vi "plane_from_3-pts.vi"(11 "Input":dbl[][](array[numeric])) -> (2 "Cross Product":dbl[](array[numeric]), 3 "gradient-out":dbl[](array[numeric]))   [LabVIEW 2024]
uses:
  <vilib>/Analysis/NI_AALPro.lvlib
panel:
  out "element":dbl
  out "In 3":dbl[](array[numeric])
  out "In 2":dbl[](array[numeric])
  out "In 1":dbl[](array[numeric])
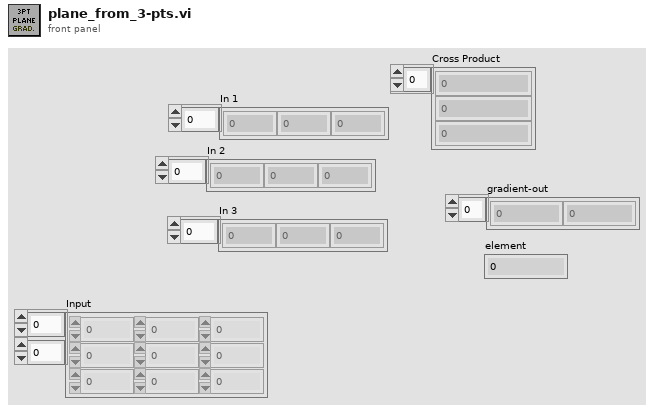
[diagram p1: front panel]
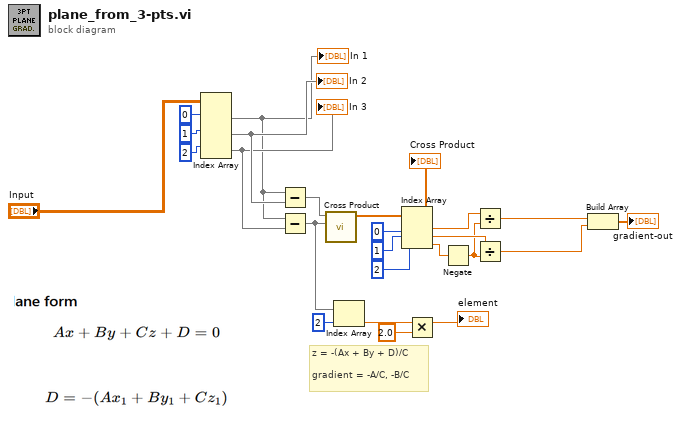
[diagram p0: block diagram]
diagram:
  # "z = -(Ax + By + D)/C\n\ngradient = -A/C, -B/C"
  n1 = Index Array(array="Input", index (row) #1=0 ("index (row)"), index (row) #2=1 ("index (row)"), index (row) #3=2 ("index (row)")) -> (element #1=w17:dbl[], element #2=w20:dbl[], element #3=w19:dbl[])  [unwired: 3 in]
  "In 1" <- w17
  "In 2" <- w20
  "In 3" <- w19
  n2 = Subtract(x=w17, y=w20) -> (x-y=w18:dbl[])
  n3 = Subtract(x=w17, y=w19) -> (x-y=w5:dbl[])
  n4 = call <vilib>:"Cross Product.vi"("B Vector"=w5, "A Vector"=w18) -> ("Cross Product"=w16:dbl[])  [unwired: 8 in, 1 out]
  "Cross Product" <- w16
  n5 = Index Array(array=w5, index=2) -> (element=w3:dbl)
  n6 = Index Array(array=w16, index #1=0 ("index (row)"), index #2=1 ("index (row)"), index #3=2 ("index (row)")) -> (element #1=w11:dbl, element #2=w12:dbl, element #3=w10:dbl)
  n7 = Multiply(x=w3, y=2.0) -> (x*y=→"element":dbl)
  n8 = Negate(x=w10) -> (-x=w9:dbl)
  n9 = Divide(x=w11, y=w9) -> (x/y=w8:dbl)
  n10 = Divide(x=w12, y=w9) -> (x/y=w7:dbl)
  n11 = Build Array(w8, w7) -> (→"gradient-out":dbl[])
